vi "insert_into_waveform.vi"(8 "timestamp":timestamp, 11 "waveform":waveform(dbl)) -> (3 "updated waveform":waveform(dbl))   [LabVIEW 2020]
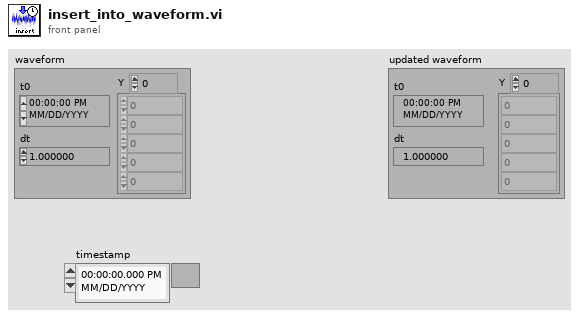
[diagram p1: front panel]
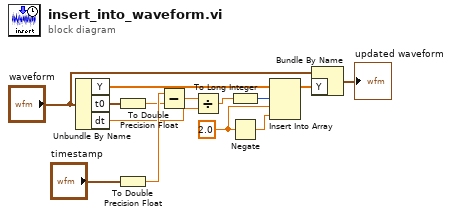
[diagram p0: block diagram]
diagram:
  w3 = 2.0 ("new element/subarray")
  n1 = Unbundle By Name("waveform") -> ("Y"=w4:dbl[], "t0"=w12:timestamp, "dt"=w7:dbl)
  n2 = To Double Precision Float(number=w12) -> (double precision float=w9:dbl)
  n3 = To Double Precision Float(number="timestamp") -> (double precision float=w10:dbl)
  n4 = Subtract(x=w10, y=w9) -> (x-y=w8:dbl)
  n5 = Divide(x=w8, y=w7) -> (x/y=w6:dbl)
  n6 = To Long Integer(number=w6) -> (32bit integer=w5:i32)
  n7 = Negate(x=w3) -> (-x=w2:dbl)
  n8 = Insert Into Array(array=w4, index=w5, new element #1=w3, new element #2=w2) -> (w1:dbl[])
  n9 = Bundle By Name(cluster="waveform", "Y"=w1) -> (→"updated waveform":waveform(dbl))
